vi "GetRoutes.vi"(8 "error in (no error)":errorcluster, 11 "reference in":refnum<class "Switch_Keysight_34934A.lvclass">) -> (0 "error out":errorcluster, 2 "Routes":T1(array[cluster]), 3 "reference in":refnum<class "Switch_Keysight_34934A.lvclass">)   [LabVIEW 2022 SP3, in "Switch_Keysight_34934A.lvlib" / "Switch_Keysight_34934A.lvclass"]
uses:
  Switch_Keysight_34934A.lvclass
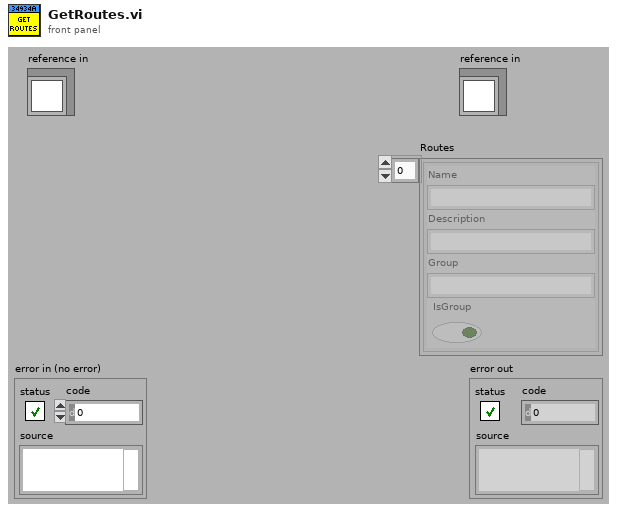
[diagram p1: front panel]
types:
  T1 = cluster{"Name":string, "Description":string, "Group":string, "IsGroup":bool}[]
  T2 = cluster{"Name":string, "Description":string, "Group":string, "IsGroup":bool}
  T3 = typedef "Switch_Keysight_34934A.lvlib/Switch_Keysight_34934A.lvclass/ObjectAttributes.ctl" = cluster{"Config":T4, "VISA ref":refnum<visa-resource-name>, "M1H":bool[][], "M2H":bool[][], "M1L":bool[][], "M2L":bool[][], "route":string, "State":bool[], "StateModBit":bool[], "UpdateEvent":refnum<user-event>}
  T4 = typedef "Switch_Keysight_34934A.lvlib/Switch_Keysight_34934A.lvclass/Config.ctl" = cluster{"VISA":refnum<visa-resource-name>, "Slot":i32, "SwitchMap":cluster{"Name":string, "Route":string[], "UnRoute":string[], "Description":string, "Group":string, "IsGroup":bool}[], "Sim":bool}
  T5 = cluster{"Name":string, "Route":string[], "UnRoute":string[], "Description":string, "Group":string, "IsGroup":bool}[]
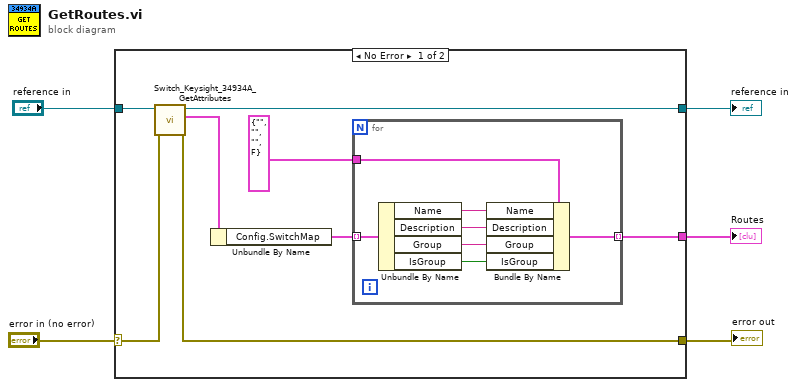
[diagram p0: block diagram]
diagram:
  n1 = case shown="No Error" "error in (no error)" {
    selector: "error in (no error)" -> [w13 w22]
    tunnel: [w11 w22] -> w4
    tunnel: [w9 w21] -> w2
    tunnel: "reference in" -> [w10 w21]
    tunnel: [w6 _] -> w1
    frame No Error {
      n2 = call "Switch_Keysight_34934A_GetAttributes.vi"("error in (no error)"=w13, "reference in"=w10) -> ("error out"=w11:errorcluster, "Data"=w12:T3, "reference out"=w9:refnum<class "Switch_Keysight_34934A.lvclass">)  [unwired: 6 in, 1 out]
      n3 = Unbundle By Name(w12) -> ("Config.SwitchMap"=w8:T5)
      n4 = for {
        tunnel: w8 -> [w19] mode=indexing
        tunnel: T2 {"Name"="", "Description"="", "Group"="", "IsGroup"=FALSE} ("Route") -> [w20]
        tunnel: [w14] -> w6 mode=indexing
        n5 = Unbundle By Name(w19) -> ("Name"=w18:string, "Description"=w17:string, "Group"=w16:string, "IsGroup"=w15:bool)
        n6 = Bundle By Name(cluster=w20, "Name"=w18, "Description"=w17, "Group"=w16, "IsGroup"=w15) -> (w14:T2)
      }
    }
    frame Error {
    }
  }
  "error out" <- w4
  "reference in" <- w2
  "Routes" <- w1
